vi "PH_StatusHandler.contents.vi"   [LabVIEW 2014, in "PH_StatusHandler.lvlib"]
doc: "This class is forseen to control black boxes (motion).\n\nThis class is part of the PHELIX device layer."
uses:
  PH_StatusHandler.lvlib
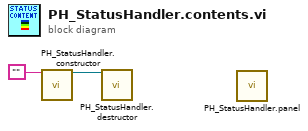
[diagram p0: block diagram]
diagram:
  n1 = call "PH_StatusHandler.constructor.vi"("name"="") -> ("i ref out"=w1:refnum<vi>)  [unwired: 16 in, 2 out]
  n2 = call "PH_StatusHandler.destructor.vi"("i ref in"=w1) -> ()  [unwired: 18 in, 1 out]
  n3 = call "PH_StatusHandler.panel.vi"() -> ()  [unwired: 19 in, 1 out]
